vi "Update Count.vi"(8 "error in (no error)":errorcluster, 10 "Count":u64, 11 "Chef UI in":refnum<class "Chef UI.lvclass">) -> (0 "error out":errorcluster, 3 "Chef UI out":refnum<class "Chef UI.lvclass">)   [LabVIEW 2024, in "Chef UI.lvlib" / "Chef UI.lvclass"]
uses:
  Chef UI.lvclass
  Chef UI.lvclass/Chef UI.ctl
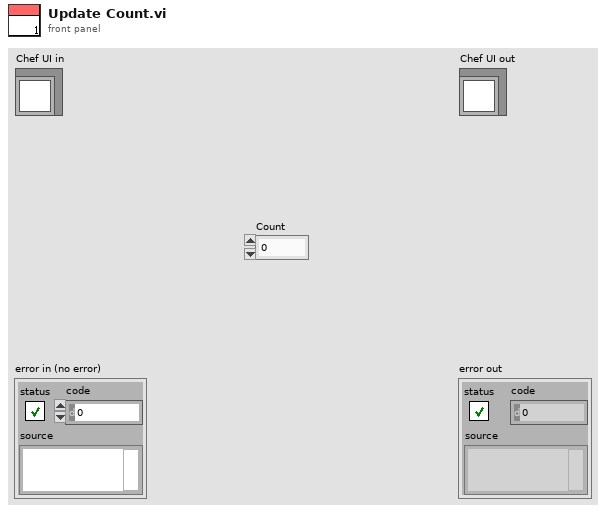
[diagram p1: front panel]
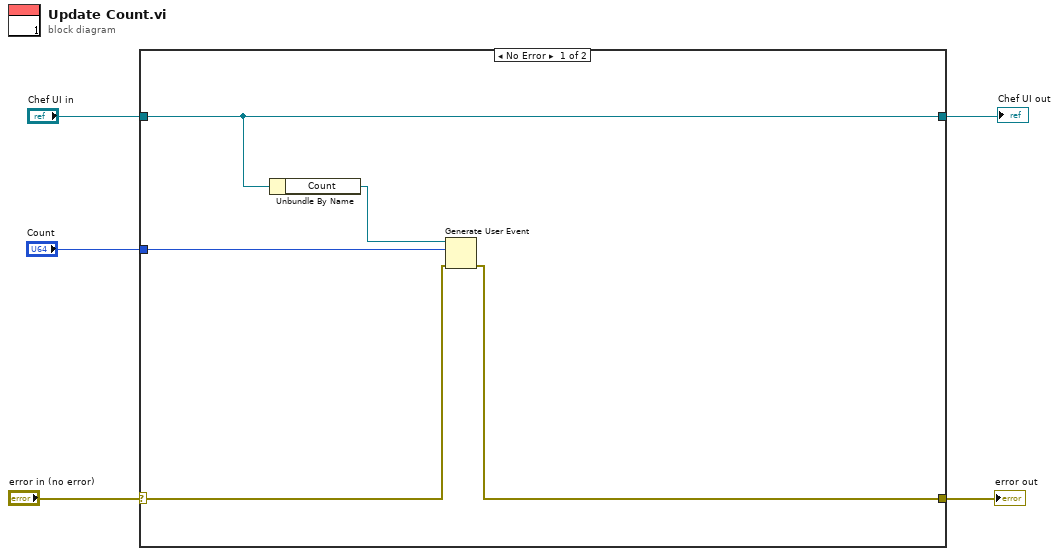
[diagram p0: block diagram]
diagram:
  n1 = case shown="No Error" "error in (no error)" {
    selector: "error in (no error)" -> [w7 w11]
    tunnel: [w6 w11] -> w4
    tunnel: "Chef UI in" -> [w10 w12]
    tunnel: [w10 w12] -> w2
    tunnel: "Count" -> [w8 _]
    frame No Error {
      n2 = Unbundle By Name(w10) -> ("Count"=w9:refnum<user-event>)
      n3 = Generate User Event(user event=w9, event data cluster=w8, error in=w7) -> (error out=w6:errorcluster)  [unwired: 1 in, 1 out]
    }
    frame Error {
    }
  }
  "error out" <- w4
  "Chef UI out" <- w2
